vi "Main_Console.vi"() -> ()   [LabVIEW 2021]
doc: "This VI is MainVI that Interact with user"
uses:
  Library/Custom_Sort_Library.lvlib
  Library/Library_Controls/Order (Z to A).ctl
panel:
  in  "Error_In":errorcluster
  out "Error_Out":errorcluster
  out "Table":string[][](table)
  in  "CSV_File_Path":path
  in  "Text_File_Path":path=path "D:/Project Git file/Assignments/Progress_Review_Coding_01/Library/text01.txt"
  in  "Save":bool
  in  "Sort":bool
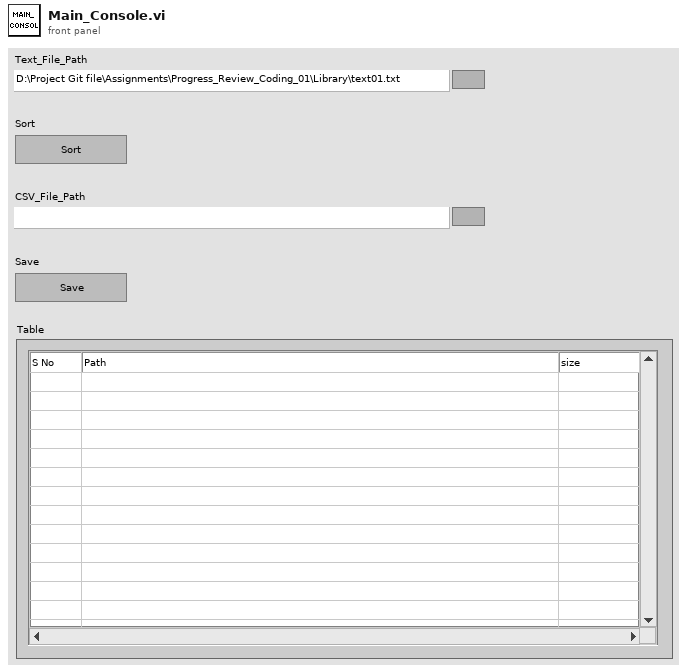
[diagram p1: front panel]
types:
  T1 = typedef "Custom_Sort_Library.lvlib/Order (Z to A).ctl" = enum16{"Z to A", "A to Z"}
  T2 = enum16{"Left Button", "Center Button", "Right Button", "Window Close"}
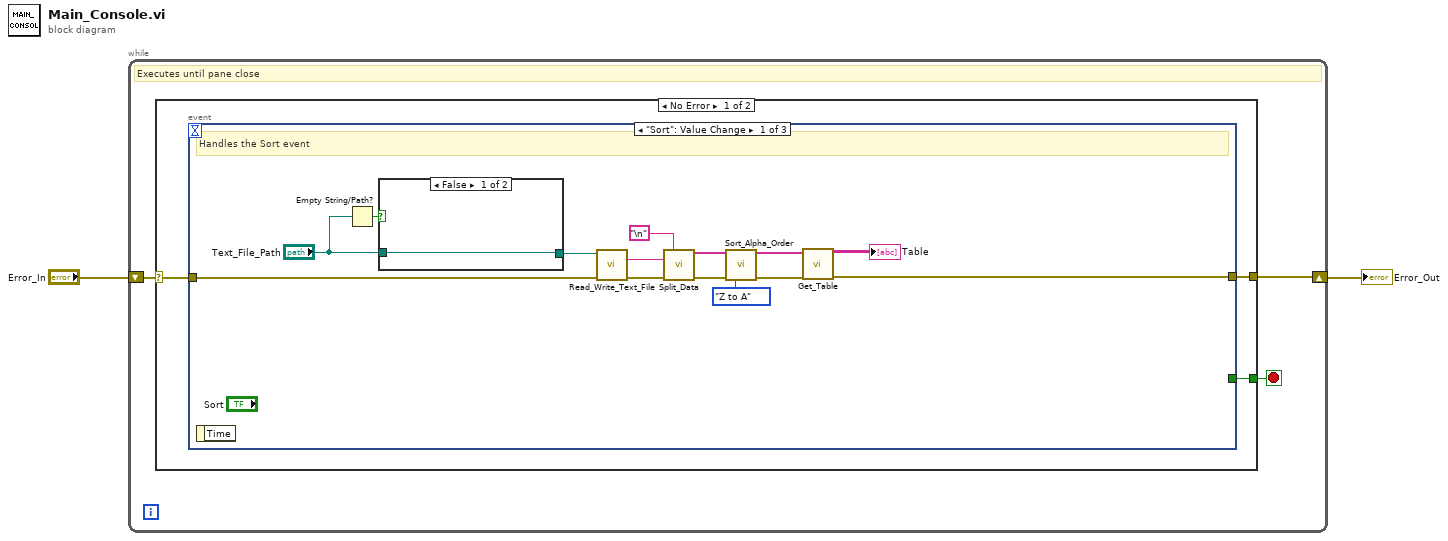
[diagram p0: block diagram]
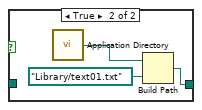
[diagram p2: hidden frame]
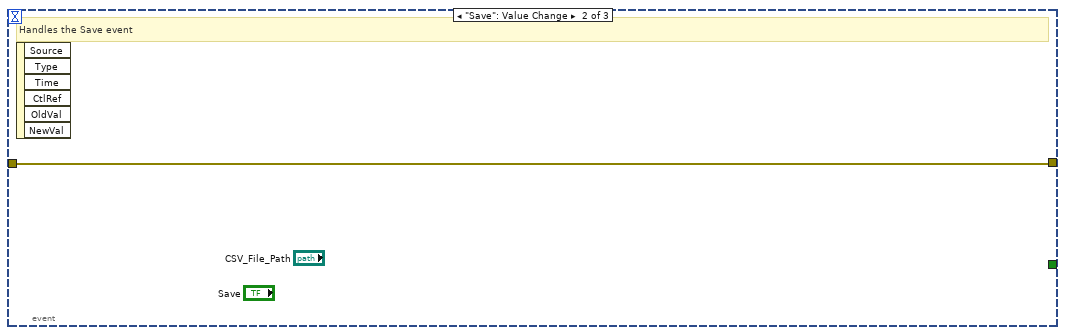
[diagram p3: hidden frame]
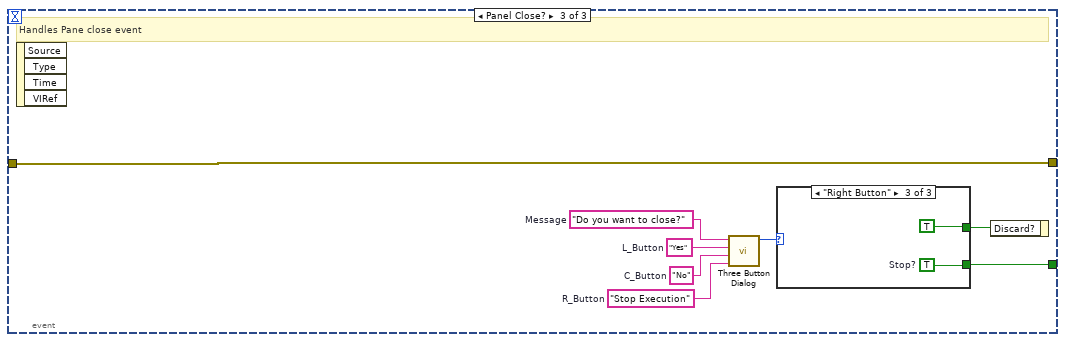
[diagram p4: hidden frame]
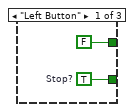
[diagram p5: hidden frame]
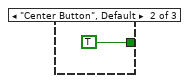
[diagram p6: hidden frame]
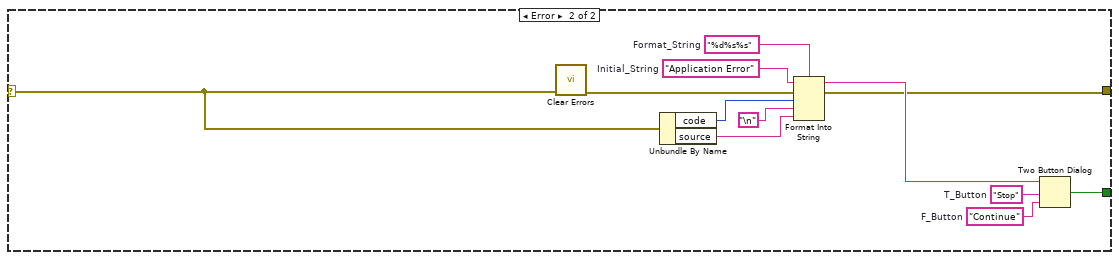
[diagram p7: hidden frame]
diagram:
  n1 = while {
    shift-right: [w4] -> w1
    shift-left: "Error_In" -> [w5]
    stop <- w3 stop-if-true
    # "Executes until pane close"
    n2 = case shown="No Error" w5 {
      selector: w5 -> [w8 w43]
      tunnel: [w7 w42] -> w4
      tunnel: [w6 w41] -> w3
      frame No Error {
        n3 = event shown="[0] \"Sort\": Value Change" {
          selector: _ -> [_ _ _]
          dyn-events: _ -> [_ _ _]
          timeout: _ -> [_ _ _]
          tunnel: w8 -> [w22 w27 w28]
          tunnel: [w12 w27 w28] -> w7
          tunnel: [_ _ w29] -> w6
          event "Sort": Value Change {
            # "Handles the Sort event"
            n4 = event-data() -> ()  [unwired: 1 in, 1 out]
            n5 = Empty String/Path?(string/path="Text_File_Path") -> (empty?=w11:bool)
            n6 = case shown="False" w11 {
              tunnel: [w23 w24] -> w10
              tunnel: "Text_File_Path" -> [w23 _]
              frame False {
              }
              frame True {
                n7 = call <vilib>:"Application Directory.vi"() -> ("Application Directory"=w26:path)
                n8 = Build Path(base path=w26, name or relative path=path "Library/text01.txt") -> (appended path=w24:path)
              }
            }
            n9 = call "Read_Write_Text_File.vi"("File_Path_In"=w10, "Error_In"=w22) -> ("Data_Out"=w19:string, "Error_Out"=w21:errorcluster)  [unwired: 11 in, 1 out]
            n10 = call "Split_Data.vi"("Delimiter"="\n", "Data_In"=w19, "Error_In"=w21) -> ("Split_Data_Out"=w17:string[], "Error_Out"=w20:errorcluster)  [unwired: 11 in]
            n11 = call "Sort_Alpha_Order.vi"("Split_Data"=w17, "Error_In"=w20, "Order (Z to A)"=Order_(Z_to_A)."Z to A") -> ("Sorted_Array"=w15:string[], "Error_Out"=w13:errorcluster)  [unwired: 11 in]
            n12 = call "Get_Table.vi"("Sorted_Array"=w15, "Error_In"=w13) -> ("Table"=→"Table":string[][], "Error_Out"=w12:errorcluster)  [unwired: 12 in]
          }
          event "Save": Value Change {
            # "Handles the Save event"
            n13 = event-data() -> ()  [unwired: 1 in, 6 out]
          }
          event Panel Close? {
            w32 = "Stop Execution"  # R_Button
            w33 = "No"  # C_Button
            w34 = "Yes"  # L_Button
            w35 = "Do you want to close?"  # Message
            # "Handles Pane close event"
            n14 = event-data() -> ()  [unwired: 1 in, 4 out]
            n15 = call <vilib>:"Three Button Dialog.vi"("Right Button Text (\"Cancel\")"=w32, "Center Button Text (\"No\")"=w33, "Left Button Text (\"Yes\")"=w34, "message"=w35) -> ("Which Button?"=w31:T2)  [unwired: 7 in]
            n16 = case shown="\"Right Button\"" w31 {
              tunnel: [FALSE TRUE TRUE] -> w30
              tunnel: [w36 _ w40] -> w29
              frame "Left Button" {
                w36 = TRUE  # Stop?
              }
              frame "Center Button", Default {
              }
              frame "Right Button" {
                w40 = TRUE  # Stop?
              }
            }
            n17 = event-data("Discard?"=w30) -> ()  [unwired: 1 in, 1 out]
          }
        }
      }
      frame Error {
        w48 = "%d%s%s"  # Format_String
        w49 = "Application Error"  # Initial_String
        w50 = "Stop"  # T_Button
        w51 = "Continue"  # F_Button
        n18 = call <vilib>:"Clear Errors.vi"("error in (no error)"=w43) -> ("error out"=w46:errorcluster)  [unwired: 5 in, 1 out]
        n19 = Unbundle By Name(w43) -> ("code"=w45:i32, "source"=w44:string)
        n20 = Format Into String(format string=w48, initial string=w49, error in=w46, w45, "\n", w44) -> (resulting string=w52:string, error out=w42:errorcluster)
        n21 = Two Button Dialog(message=w52, 1:w51, 2:w50) -> (T button?=w41:bool)
      }
    }
  }
  "Error_Out" <- w1
